vi "save_adc_reg_cfg.vi"(9 "filename_cfg":string, 10 "ADC in":u32[](array[numeric]), 11 "ADC in":u32[](array[numeric])) -> ()   [LabVIEW 2015]
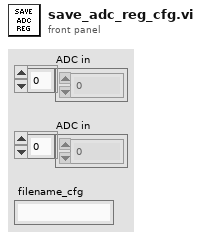
[diagram p1: front panel]
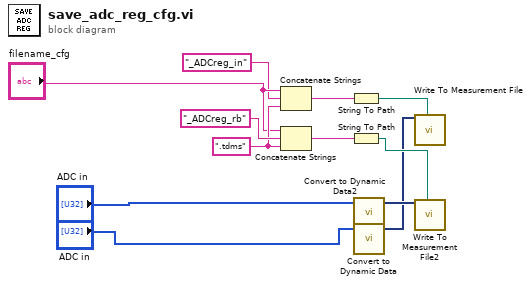
[diagram p0: block diagram]
diagram:
  w9 = ".tdms" ("string")
  n1 = Concatenate Strings("filename_cfg", "_ADCreg_in" ("string"), w9) -> (w3:string)
  n2 = Concatenate Strings("filename_cfg", "_ADCreg_rb" ("string"), w9) -> (w11:string)
  n3 = String To Path(string=w3) -> (path=w4:path)
  n4 = String To Path(string=w11) -> (path=w12:path)
  n5 = call "Convert to Dynamic Data2"("Array"="ADC in") -> ("Dynamic Data Type"=w7:dynamicdata)  [unwired: 3 in]
  n6 = call "Convert to Dynamic Data"("Array"="ADC in") -> ("Dynamic Data Type"=w2:dynamicdata)  [unwired: 3 in]
  n7 = call "Write To Measurement File"("Signals"=w2, "Filename"=w4) -> ()  [unwired: 15 in, 3 out]
  n8 = call "Write To Measurement File2"("Signals"=w7, "Filename"=w12) -> ()  [unwired: 15 in, 3 out]
